vi "exercicio8_despertador.vi"() -> ()   [LabVIEW 2018]
panel:
  in  "?":bool
  in  "?":bool
  out "Hora Atual":string
  out "Boolean":bool
  in  "Minutos":string
  in  "Hora 24h":string
  # ":"
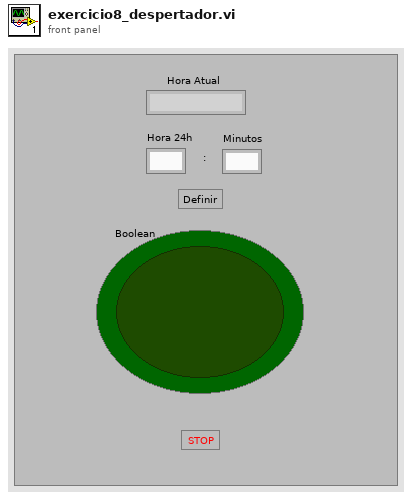
[diagram p1: front panel]
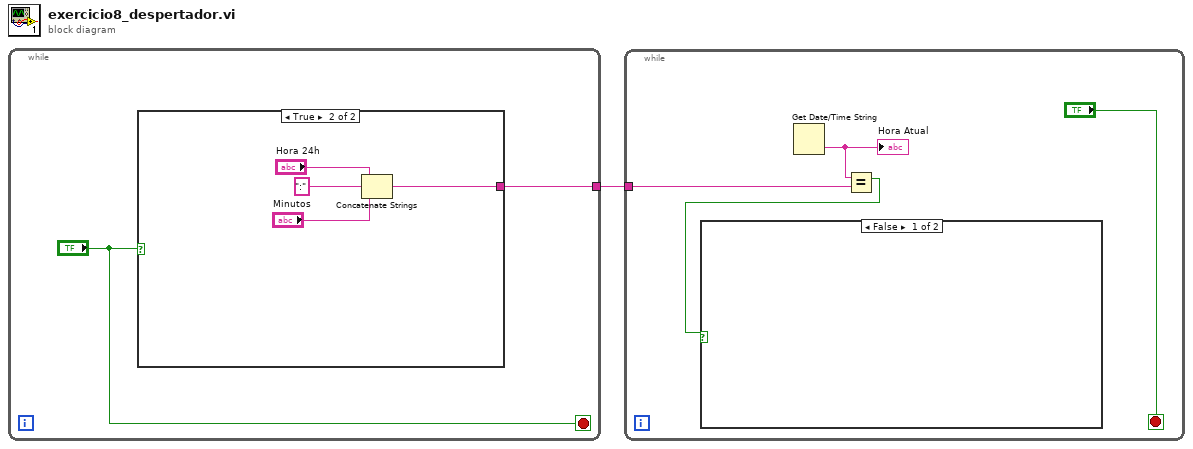
[diagram p0: block diagram]
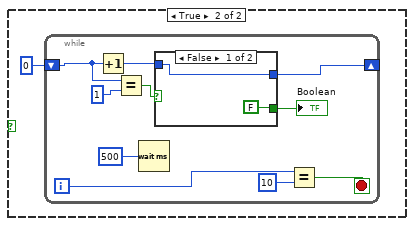
[diagram p2: hidden frame]
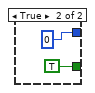
[diagram p3: hidden frame]
diagram:
  n1 = while {
    tunnel: [w2] -> w1
    stop <- "?" stop-if-true
    n2 = case shown="True" "?" {
      tunnel: [_ w4] -> w2
      frame False {
      }
      frame True {
        n3 = Concatenate Strings("Hora 24h", ":" ("string"), "Minutos") -> (w4:string)
      }
    }
  }
  n4 = while {
    tunnel: w1 -> [w8]
    stop <- "?" stop-if-true
    n5 = Get Date/Time String() -> (time string=w11:string)  [unwired: 3 in, 1 out]
    "Hora Atual" <- w11
    n6 = Equal?(x=w11, y=w8) -> (x = y?=w9:bool)
    n7 = case shown="False" w9 {
      frame False {
      }
      frame True {
        n8 = while {
          shift-right: [w21] -> _
          shift-left: 0 -> [w14]
          i -> [w19]
          stop <- w17 stop-if-true
          n9 = Increment(x=w14) -> (x+1=w22:i32)
          n10 = Equal?(x=w14, y=1) -> (x = y?=w15:bool)
          n11 = Wait (ms)(milliseconds to wait=u32 500) -> ()  [unwired: 1 out]
          n12 = case shown="False" w15 {
            tunnel: w22 -> [w24 _]
            tunnel: [w24 0] -> w21
            tunnel: [FALSE TRUE] -> w20
            frame False {
            }
            frame True {
            }
          }
          "Boolean" <- w20
          n13 = Equal?(x=w19, y=10) -> (x = y?=w17:bool)
        }
      }
    }
  }
